vi "niFpgaFFTMemWriteLogic.vi"(0 "x from bf":T3 {"Real" format="%.16g"; "Imaginary" format="%.16g"}, 2 "input data":T3 {"Real" format="%.16g"; "Imaginary" format="%.16g"}, 5 "y from bf":T3 {"Real" format="%.16g"; "Imaginary" format="%.16g"}, 7 "read address":u16, 9 "enable mem":bool, 12 "control signals":T2) -> (4 "memory output A":T1 {"data"."Real" format="%.16g"; "data"."Imaginary" format="%.16g"}, 6 "memory output B":T1 {"data"."Real" format="%.16g"; "data"."Imaginary" format="%.16g"})   [LabVIEW 2017]
uses:
  <vilib>/rvi/Analysis/measure/FFT/templates/niFPGA FFT Control Signals.ctl
  <vilib>/rvi/FXPMathLib/basic elements/FxpDiscreteDelay/XNode/nifxpmath_DiscreteDelay.xnode
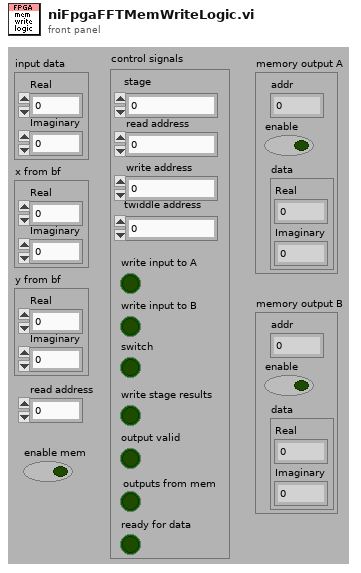
[diagram p1: front panel]
types:
  T1 = cluster{"addr":u16, "enable":bool, "data":cluster{"Real":fxp<+/-,16,1>, "Imaginary":fxp<+/-,16,1>}}
  T2 = typedef "niFPGA FFT Control Signals.ctl" = cluster{"read address":u16, "switch":bool, "write input to B":bool, "write stage results":bool, "write input to A":bool, "output valid":bool, "twiddle address":u16, "write address":u16, "outputs from mem":bool, "ready for data":bool, "stage":u8}
  T3 = cluster{"Real":fxp<+/-,16,1>, "Imaginary":fxp<+/-,16,1>}
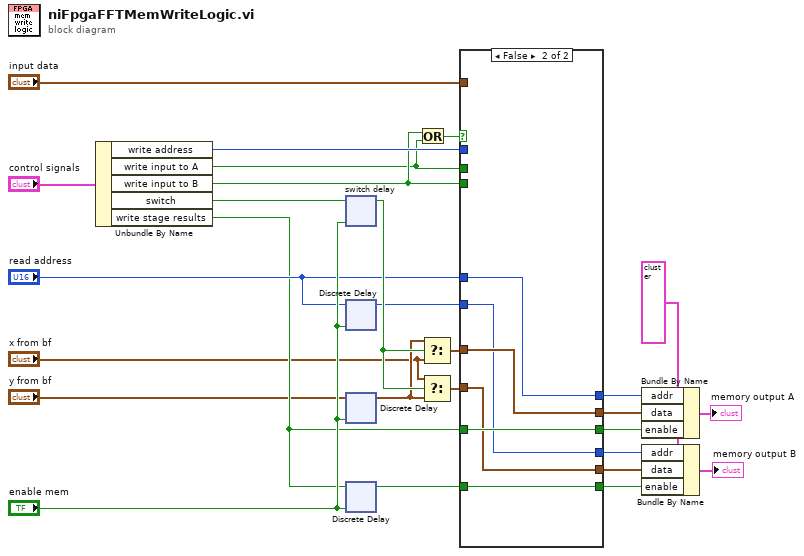
[diagram p0: block diagram]
diagram:
  w19 = T1 {"addr"=0, "enable"=FALSE, "data"={"Real"=0.0, "Imaginary"=0.0}} ("mem write cluster")
  n1 = Unbundle By Name("control signals") -> ("write address"=w23:u16, "write input to A"=w15:bool, "write input to B"=w16:bool, "switch"=w18:bool, "write stage results"=w7:bool)
  n2 = xnode ("switch delay")("D"=w18, "enable"="enable mem") -> ("Q"=w14:bool)
  n3 = xnode ("Discrete Delay")("D"="read address", "enable"="enable mem") -> ("Q"=w9:u16)
  n4 = xnode ("Discrete Delay")("D"="y from bf", "enable"="enable mem") -> ("Q"=w8:T3)
  n5 = xnode ("Discrete Delay")("D"=w7, "enable"="enable mem") -> ("Q"=w6:bool)
  n6 = Or(x=w16, y=w15) -> (x .or. y?=w17:bool)
  n7 = Select(t=w8, s=w14, f="x from bf") -> (s? t:f=w11:T3)
  n8 = Select(t="x from bf", s=w14, f=w8) -> (s? t:f=w12:T3)
  n9 = case shown="False" w17 {
    tunnel: "read address" -> [_ w35]
    tunnel: w9 -> [_ w33]
    tunnel: w12 -> [_ w32]
    tunnel: w11 -> [_ w34]
    tunnel: w7 -> [_ w37]
    tunnel: w6 -> [_ w36]
    tunnel: [w28 w34] -> w26
    tunnel: [w30 w35] -> w25
    tunnel: [w30 w33] -> w22
    tunnel: [w28 w32] -> w21
    tunnel: w15 -> [w29 _]
    tunnel: w16 -> [w31 _]
    tunnel: w23 -> [w30 _]
    tunnel: [w29 w37] -> w27
    tunnel: [w31 w36] -> w20
    tunnel: "input data" -> [w28 _]
    frame True {
    }
    frame False {
    }
  }
  n10 = Bundle By Name(cluster=w19, "addr"=w25, "data"=w26, "enable"=w27) -> (→"memory output A":T1)
  n11 = Bundle By Name(cluster=w19, "addr"=w22, "data"=w21, "enable"=w20) -> (→"memory output B":T1)
